vi "String Keyword Finder.vi"(4 "Exact Match?":bool=TRUE, 5 "Keyword List":string[](array[string]), 8 "Input String":string) -> (3 "Match?":bool)   [LabVIEW 2018]
doc: "Searches the Input String for the occurrence of at least one keyword. Also returns the number of instances found for each keyword."
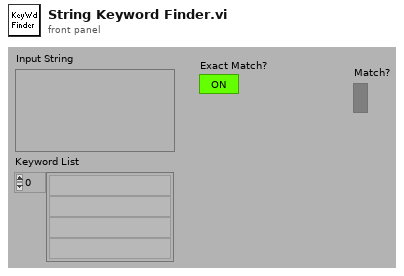
[diagram p1: front panel]
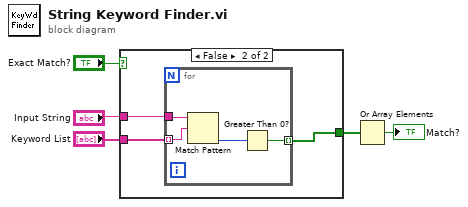
[diagram p0: block diagram]
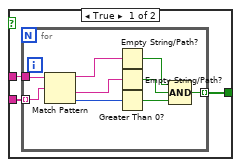
[diagram p2: hidden frame]
diagram:
  n1 = case shown="False" "Exact Match?" {
    tunnel: "Input String" -> [w8 w20]
    tunnel: "Keyword List" -> [w7 w19]
    tunnel: [w6 w18] -> w1
    frame True {
      n2 = for {
        tunnel: w7 -> [w16] mode=indexing
        tunnel: w8 -> [w17]
        tunnel: [w9] -> w6 mode=indexing
        n3 = Match Pattern(string=w17, regular expression=w16) -> (before substring=w15:string, after substring=w14:string, offset past match=w13:i32)  [unwired: 1 in, 1 out]
        n4 = Empty String/Path?(string/path=w15) -> (empty?=w12:bool)
        n5 = Empty String/Path?(string/path=w14) -> (empty?=w11:bool)
        n6 = Greater Than 0?(x=w13) -> (x > 0?=w10:bool)
        n7 = Compound Arithmetic op=AND(w12, w11, w10) -> (w9:bool)
      }
    }
    frame False {
      n8 = for {
        tunnel: w19 -> [w23] mode=indexing
        tunnel: w20 -> [w24]
        tunnel: [w21] -> w18 mode=indexing
        n9 = Match Pattern(string=w24, regular expression=w23) -> (offset past match=w22:i32)  [unwired: 1 in, 3 out]
        n10 = Greater Than 0?(x=w22) -> (x > 0?=w21:bool)
      }
    }
  }
  n11 = Or Array Elements(Boolean array=w1) -> (logical OR=→"Match?":bool)
